vi "run_event.vi"() -> ()   [LabVIEW 2011]
panel:
  out "Sent data":string
  out "Current Time":string
  in  "A225 Window":enum32{"open", "close"}(radio)
  in  "?":bool
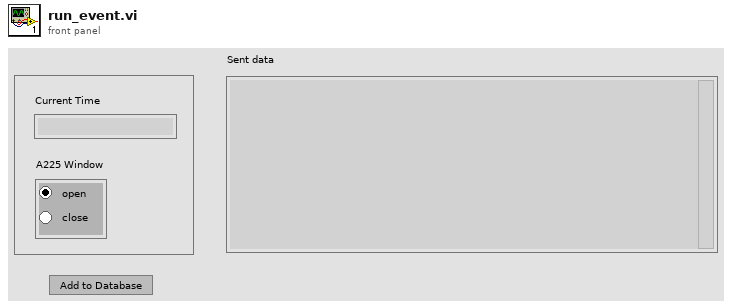
[diagram p1: front panel]
types:
  T1 = cluster{string, string, string, string, string, string}
  T2 = cluster{string, string, string, string, "date/time string":string, string}
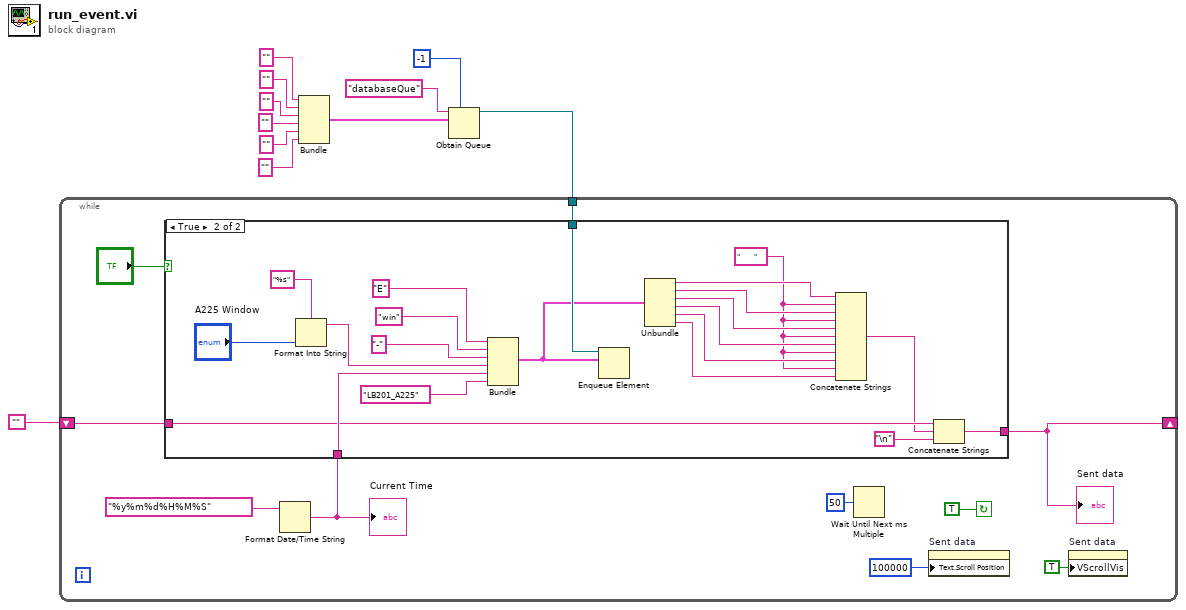
[diagram p0: block diagram]
diagram:
  n1 = Bundle("", "", "", "", "", "") -> (w8:T1)  [unwired: 1 in]
  n2 = Obtain Queue(max queue size (-1, unlimited)=-1, name (unnamed)="databaseQue", element data type=w8) -> (queue out=w2:refnum<queue>)  [unwired: 2 in, 2 out]
  n3 = while {
    tunnel: w2 -> [w19]
    shift-right: [w14] -> _
    shift-left: "" -> [w15]
    stop <- TRUE continue-if-true
    n4 = Format Date/Time String(time format string (%c)="%y%m%d%H%M%S") -> (date/time string=w16:string)  [unwired: 2 in]
    "Current Time" <- w16
    n5 = case shown="True" "?" {
      tunnel: w19 -> [_ w43]
      tunnel: w16 -> [_ w38]
      tunnel: [w22 w26] -> w14
      tunnel: w15 -> [w22 w25]
      frame False {
      }
      frame True {
        w31 = "       "
        n6 = Format Into String(format string="%s", "A225 Window") -> (resulting string=w27:string)  [unwired: 2 in, 1 out]
        n7 = Bundle("E", "win", "-", w27, "date/time string"=w38, "LB201_A225") -> (w30:T2)  [unwired: 1 in]
        n8 = Enqueue Element(queue=w43, element=w30) -> ()  [unwired: 2 in, 3 out]
        n9 = Unbundle(w30) -> (w37:string, w36:string, w35:string, w34:string, "date/time string"=w33:string, w32:string)
        n10 = Concatenate Strings(w37, w31, w36, w31, w35, w31, w34, w31, w33, w31, w32) -> (w24:string)
        n11 = Concatenate Strings(w25, w24, "\n") -> (w26:string)
      }
    }
    "Sent data" <- w14
    n12 = Wait Until Next ms Multiple(millisecond multiple=u32 50) -> ()  [unwired: 1 out]
    n13 = property on="Sent data" class="Str"("Text.Scroll Position"=u32 100000) -> ()  [unwired: 2 in, 2 out]
    n14 = property on="Sent data" class="Str"("VScrollVis"=TRUE ("Vertical Scrollbar Visible")) -> ()  [unwired: 2 in, 2 out]
  }
